vi "GetText.vi"(8 "error in (no error)":errorcluster, 10 "MenuItem":refnum<class "MGI_MenuItem.lvclass">, 11 "Menu in":refnum<class "MGI_ToolStrip.lvclass">) -> (0 "error out":errorcluster, 2 "Text":string, 3 "Menu out":refnum<class "MGI_ToolStrip.lvclass">)   [LabVIEW 2019, in "MGI_ToolStrip.lvclass"]
doc: "Gets the Text of the Menu Item. Required to be overridden.\n\nAuthored by Derek E. Trepanier\nsupport@mooregoodideas.com\nwww.mooregoodideas.com\n\nCopyright (c) 2012, Moore Good Ideas, Inc.\n\nAll rights reserved.\n\nRedistribution and use in source and binary forms, with or without modification, are permitted provided that the following conditions are met:\n\n * Redistributions of source code must retain the above copyright notice, this list of conditions and the following disclaimer.\n * Redistributions in binary form must reproduce the above copyright notice, this list of conditions and the following disclaimer in the documentation and/or other materials provided with the distribution.\n * Neither the name of Moore Good Ideas, Inc. nor the names of its contributors may be used to endorse or promote products derived from this software without specific prior written permission.\n\nTHIS SOFTWARE IS PROVIDED BY THE COPYRIGHT HOLDERS AND CONTRIBUTORS \"AS IS\" AND ANY EXPRESS OR IMPLIED WARRANTIES, INCLUDING, BUT NOT LIMITED TO, THE IMPLIED WARRANTIES OF MERCHANTABILITY AND FITNESS FOR A PARTICULAR PURPOSE ARE DISCLAIMED. IN NO EVENT SHALL THE COPYRIGHT OWNER OR CONTRIBUTORS BE LIABLE FOR ANY DIRECT, INDIRECT, INCIDENTAL, SPECIAL, EXEMPLARY, OR CONSEQUENTIAL DAMAGES (INCLUDING, BUT NOT LIMITED TO, PROCUREMENT OF SUBSTITUTE GOODS OR SERVICES; LOSS OF USE, DATA, OR PROFITS; OR BUSINESS INTERRUPTION) HOWEVER CAUSED AND ON ANY THEORY OF LIABILITY, WHETHER IN CONTRACT, STRICT LIABILITY, OR TORT (INCLUDING NEGLIGENCE OR OTHERWISE) ARISING IN ANY WAY OUT OF THE USE OF THIS SOFTWARE, EVEN IF ADVISED OF THE POSSIBILITY OF SUCH DAMAGE."
uses:
  MGI_ToolStrip.lvclass
  <userlib>/_MGI/Menu Building/MenuItem/MGI_MenuItem.lvclass
  System.Windows.Forms
  <userlib>/_MGI/Menu Building/MenuItem/Read Full Tag.vi
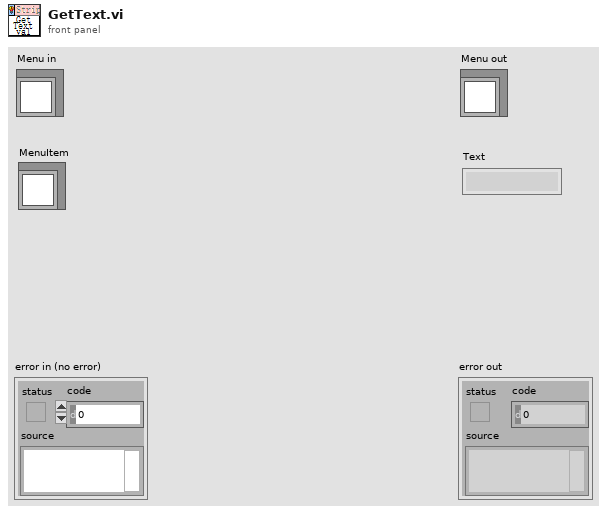
[diagram p1: front panel]
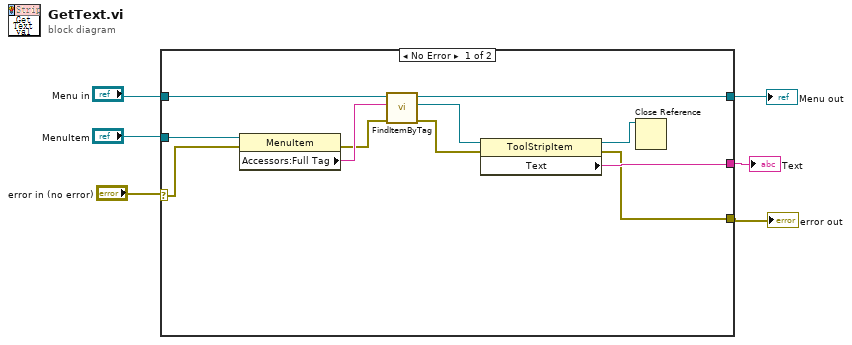
[diagram p0: block diagram]
diagram:
  n1 = case shown="No Error" "error in (no error)" {
    selector: "error in (no error)" -> [w15 w18]
    tunnel: "Menu in" -> [w14 w19]
    tunnel: [w13 w19] -> w3
    tunnel: [w7 w18] -> w4
    tunnel: "MenuItem" -> [w16 _]
    tunnel: [w8 _] -> w2
    frame No Error {
      n2 = property class="MenuItem"(reference=w16, error in=w15) -> (error out=w11:errorcluster, "Accessors:Full Tag"=w12:string)  [unwired: 1 out]
      n3 = call "FindItemByTag.vi"("error in (no error)"=w11, "Tag"=w12, "MGI_ToolStrip in"=w14) -> ("error out"=w9:errorcluster, "ToolStripItem"=w10:refnum<k24>, "MGI_ToolStrip out"=w13:refnum<class "MGI_ToolStrip.lvclass">)  [unwired: 6 in]
      n4 = property class="ToolStripItem"(reference=w10, error in=w9) -> (reference out=w17:refnum<k24>, error out=w7:errorcluster, "Text"=w8:string)
      n5 = Close Reference(reference=w17) -> ()  [unwired: 1 in, 1 out]
    }
    frame Error {
    }
  }
  "error out" <- w4
  "Menu out" <- w3
  "Text" <- w2
